vi "save DB after move.vi"(7 "Position (units) in":dbl, 8 "error in (no error)":errorcluster, 9 "Axis":i32, 10 "VISA resource name out in":refnum<visa-resource-name>, 11 "ESP302 in":refnum<class "ESP302.lvclass">) -> (0 "error out":errorcluster, 1 "Axis Status":T1(ring), 2 "VISA resource name out out":refnum<visa-resource-name>, 3 "ESP302 out":refnum<class "ESP302.lvclass">, 4 "Position (units) out":dbl)   [LabVIEW 2020, in "ESP302.lvclass"]
uses:
  ESP302/ESP302.lvclass
  ESP302/ESP302.lvclass/ESP302.ctl
  activeflag.ctl
  shared/OnOffTypeDef.ctl
  shared/CompressAndUpdate(Poly)/CompressAndUpdate(Enum).vi
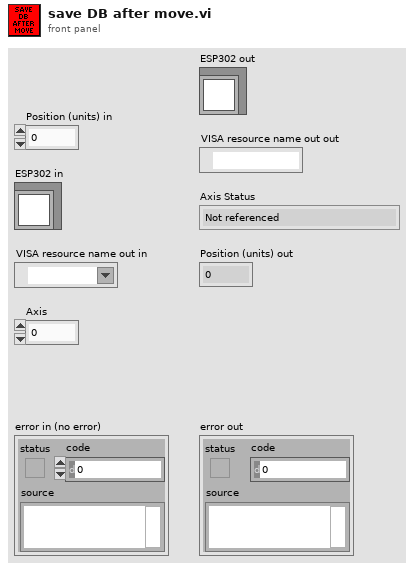
[diagram p1: front panel]
types:
  T1 = enum16{"Not referenced", "Homing", "Moving", "Ready"}
  T2 = typedef "activeflag.ctl" = enum16{"on", "off", "n/a"}
  T3 = typedef "OnOffTypeDef.ctl" = enum16{"off", "on"}
  T4 = typedef "ESP301.lvclass/SettingsTypdef.ctl" = cluster{"devport":string, "Position":cluster{"Axis 1":cluster{"Value":dbl, "Min":dbl, "Max":dbl, "StepSize":dbl, "Tolerance":dbl, "ValueActual":dbl}, "Axis 2":cluster{"Value":dbl, "Min":dbl, "Max":dbl, "StepSize":dbl, "Tolerance":dbl, "ValueActual":dbl}, "Axis 3":cluster{"Value":dbl, "Min":dbl, "Max":dbl, "StepSize":dbl, "Tolerance":dbl, "ValueActual":dbl}}, "Power":cluster{"Axis 1":T3, "Axis 2":T3, "Axis 3":T3}, "Status":cluster{"Axis 1":T5, "Axis 2":T5, "Axis 3":T5}, "Backlash":cluster{"Axis 1":cluster{"Value":dbl, "Min":dbl, "Max":dbl, "StepSize":dbl, "Tolerance":dbl, "ValueActual":dbl}, "Axis 2":cluster{"Value":dbl, "Min":dbl, "Max":dbl, "StepSize":dbl, "Tolerance":dbl, "ValueActual":dbl}, "Axis 3":cluster{"Value":dbl, "Min":dbl, "Max":dbl, "StepSize":dbl, "Tolerance":dbl, "ValueActual":dbl}}, "Home":cluster{"Axis 1":cluster{"Value":dbl, "Min":dbl, "Max":dbl, "StepSize":dbl, "Tolerance":dbl, "ValueActual":dbl}, "Axis 2":cluster{"Value":dbl, "Min":dbl, "Max":dbl, "StepSize":dbl, "Tolerance":dbl, "ValueActual":dbl}, "Axis 3":cluster{"Value":dbl, "Min":dbl, "Max":dbl, "StepSize":dbl, "Tolerance":dbl, "ValueActual":dbl}}, "MoveToHardLimit":cluster{"Axis 1":T6, "Axis 2":T6, "Axis 3":T6}, "relativeMove":cluster{"Axis 1neg":T3, "Axis 2neg":T3, "Axis 3neg":T3, "Axis 1pos":T3, "Axis 2pos":T3, "Axis 3pos":T3}, "stepsize":cluster{"Value":dbl, "Min":dbl, "Max":dbl, "StepSize":dbl, "Tolerance":dbl, "ValueActual":dbl}, "automotoroff":T3, "ResetBeforeMove":T3, "Enable":cluster{"Axis 1":T3, "Axis 2":T3, "Axis 3":T3}, "InitWithDBValues":T3}
  T5 = typedef "status_TypDef.ctl" = enum16{"Not referenced", "Homing", "Moving", "Ready"}
  T6 = typedef "Hardware limit.ctl" = enum16{"pos", "neg"}
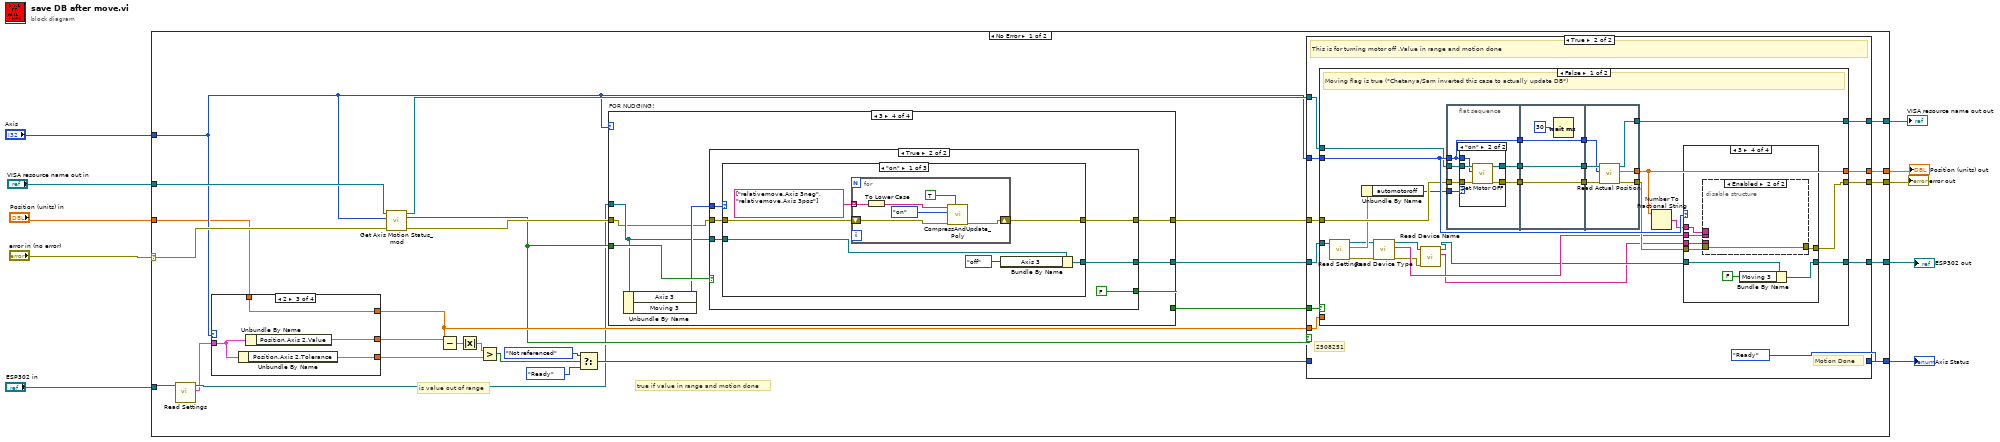
[diagram p0: block diagram]
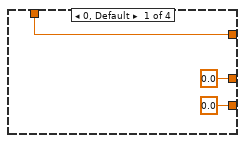
[diagram p2: hidden frame]
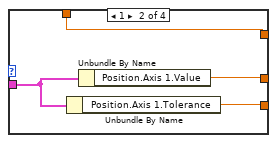
[diagram p3: hidden frame]
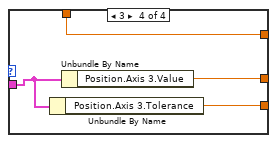
[diagram p4: hidden frame]
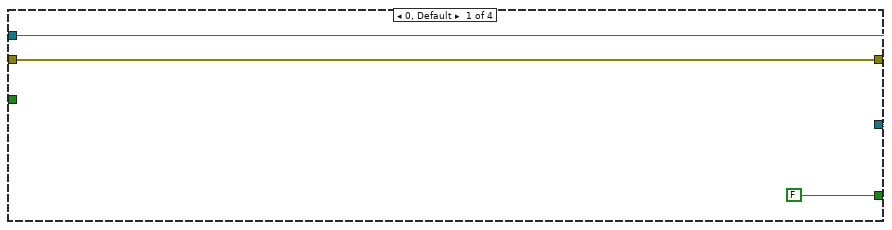
[diagram p5: hidden frame]
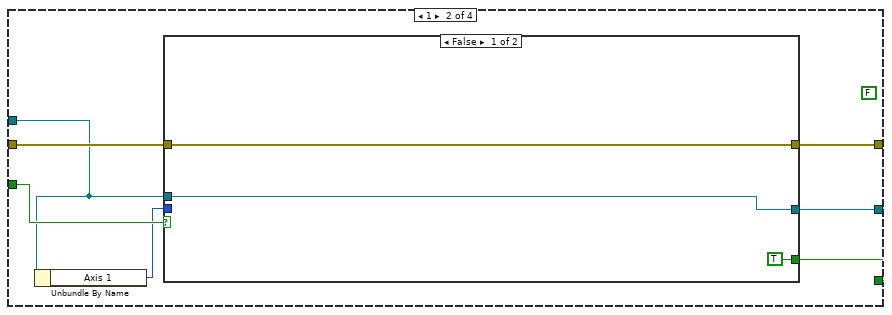
[diagram p6: hidden frame]
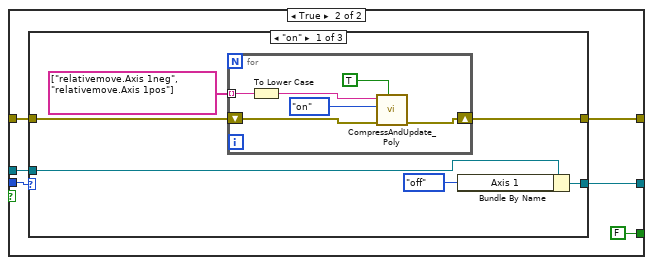
[diagram p7: hidden frame]
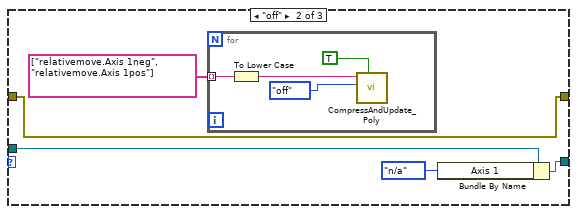
[diagram p8: hidden frame]
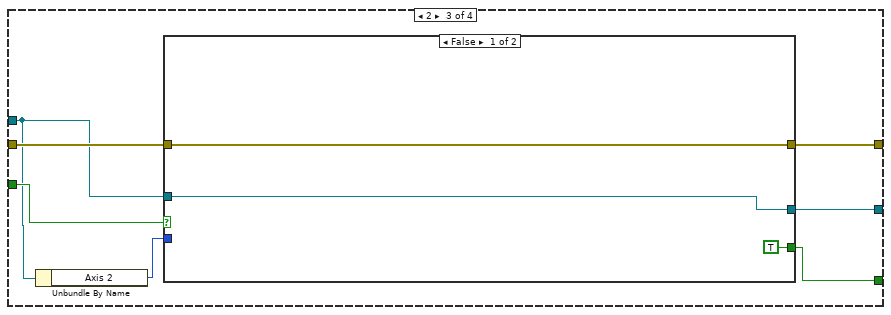
[diagram p10: hidden frame]
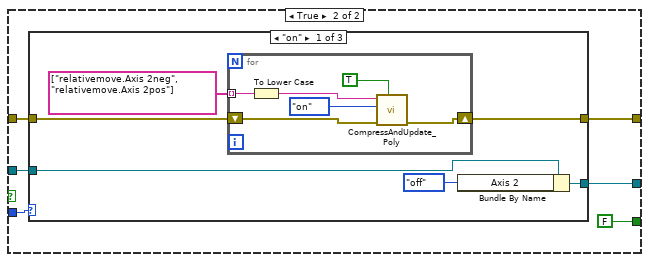
[diagram p11: hidden frame]
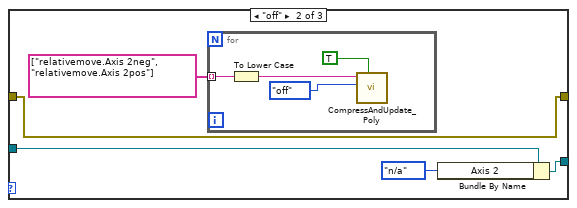
[diagram p12: hidden frame]
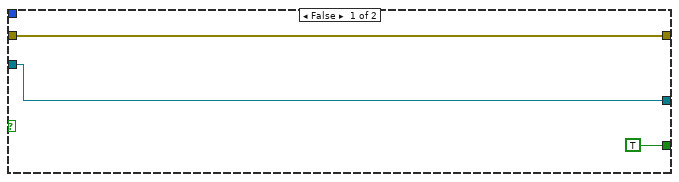
[diagram p14: hidden frame]
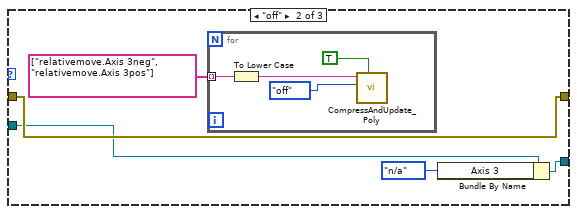
[diagram p15: hidden frame]
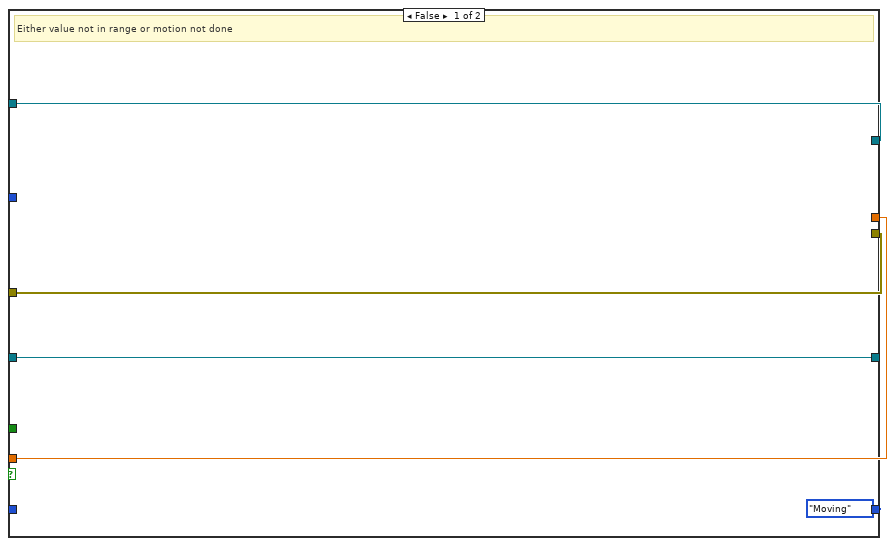
[diagram p17: hidden frame]
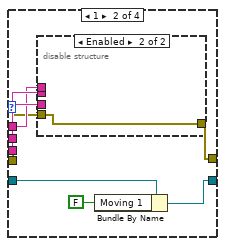
[diagram p20: hidden frame]
diagram:
  n1 = case shown="No Error" "error in (no error)" {
    selector: "error in (no error)" -> [w17 w288]
    tunnel: [w37 _] -> w4
    tunnel: [w36 w290] -> w3
    tunnel: [w35 _] -> w1
    tunnel: [w32 w289] -> w2
    tunnel: [w31 w288] -> w5
    tunnel: "ESP302 in" -> [w13 w289]
    tunnel: "VISA resource name out in" -> [w18 w290]
    tunnel: "Axis" -> [w16 _]
    tunnel: "Position (units) in" -> [w15 _]
    frame No Error {
      # "true if value in range and motion done"
      # "is value out of range"
      # "2508251"
      n2 = call-dynamic "Read Settings.vi"("ESP301 in"=w13) -> ("Settings"=w11:T4, "ESP301 out"=w14:refnum<class "ESP302.lvclass">)  [unwired: 8 in, 1 out]
      n3 = case shown="2" w16 {
        tunnel: [0.0 ("Tolerance") w44 w47 w51] -> w24
        tunnel: [0.0 ("Value") w43 w48 w52] -> w25
        tunnel: [w38 w42 w46 w50] -> w20
        tunnel: w15 -> [w38 w42 w46 w50]
        tunnel: w11 -> [_ w41 w45 w49]
        frame 0, Default {
        }
        frame 1 {
          n4 = Unbundle By Name(w41) -> ("Position.Axis 1.Tolerance"=w44:dbl)
          n5 = Unbundle By Name(w41) -> ("Position.Axis 1.Value"=w43:dbl)
        }
        frame 2 {
          n6 = Unbundle By Name(w45) -> ("Position.Axis 2.Tolerance"=w47:dbl)
          n7 = Unbundle By Name(w45) -> ("Position.Axis 2.Value"=w48:dbl)
        }
        frame 3 {
          n8 = Unbundle By Name(w49) -> ("Position.Axis 3.Tolerance"=w51:dbl)
          n9 = Unbundle By Name(w49) -> ("Position.Axis 3.Value"=w52:dbl)
        }
      }
      n10 = call "Get Axis Motion Status_mod.vi"("error in (no error)"=w17, "Axis (1)"=w16, "VISA resource name"=w18) -> ("error out"=w21:errorcluster, "Motion Done"=w19:bool, "VISA resource name out"=w23:refnum<visa-resource-name>)  [unwired: 2 in]
      n11 = Subtract(x=w25, y=w20) -> (x-y=w28:dbl)
      n12 = Absolute Value(x=w28) -> (abs(x)=w30:dbl)
      n13 = Greater?(x=w30, y=w24) -> (0:w26:bool)
      n14 = Select(t=T1."Not referenced" ("Axis 3"), s=w26, f=T1."Ready" ("Axis 3")) -> (s? t:f=w27:T1)
      n15 = case "FOR NUDGING!" shown="3" w16 {
        tunnel: w14 -> [w53 w58 w97 w136]
        tunnel: [FALSE ("Moving 3") w56 w95 w134] -> w34
        tunnel: w19 -> [_ w62 w101 w140]
        tunnel: [w53 w57 w96 w138] -> w33
        tunnel: w21 -> [w54 w60 w100 w135]
        tunnel: [w54 w59 w99 w139] -> w22
        frame 0, Default {
        }
        frame 1 {
          (unwired) FALSE ("Moving 2")
          n16 = Unbundle By Name(w58) -> ("Axis 1"=w61:T2)
          n17 = case shown="False" w62 {
            tunnel: [w65 w71] -> w57
            tunnel: [w64 w70] -> w59
            tunnel: w60 -> [w64 w69]
            tunnel: w58 -> [w65 w68]
            tunnel: w61 -> [_ w67]
            tunnel: [TRUE ("Moving 2") FALSE ("Moving 2")] -> w56
            frame False {
            }
            frame True {
              n18 = case shown="\"on\"" w67 {
                tunnel: [w76 w87 w93] -> w71
                tunnel: [w72 w84 w94] -> w70
                tunnel: w69 -> [w73 w84 w94]
                tunnel: w68 -> [w74 w85 w93]
                frame "on" {
                  n19 = for {
                    tunnel: string[] ["relativemove.Axis 1neg", "relativemove.Axis 1pos"] -> [w80] mode=indexing
                    shift-right: [w78] -> w72
                    shift-left: w73 -> [w79]
                    n20 = To Lower Case(string=w80) -> (all lower case string=w82:string)
                    n21 = call-poly "CompressAndUpdate_Poly.vi"("force CVT update (false)"=TRUE, "error in"=w79, "enum variant"=OnOffTypeDef."on" ("Axis 1neg"), "command or variable name"=w82) -> ("error out"=w78:errorcluster)  [unwired: 7 in]
                  }
                  n22 = Bundle By Name(cluster=w74, "Axis 1"=activeflag."off" ("ActiveFlag")) -> (w76:refnum<class "ESP302.lvclass">)
                }
                frame "off" {
                  n23 = for {
                    tunnel: string[] ["relativemove.Axis 1neg", "relativemove.Axis 1pos"] -> [w89] mode=indexing
                    n24 = To Lower Case(string=w89) -> (all lower case string=w91:string)
                    n25 = call-poly "CompressAndUpdate_Poly.vi"("force CVT update (false)"=TRUE, "enum variant"=OnOffTypeDef."off" ("Axis 1neg"), "command or variable name"=w91) -> ()  [unwired: 8 in, 1 out]
                  }
                  n26 = Bundle By Name(cluster=w85, "Axis 1"=activeflag."n/a" ("ActiveFlag")) -> (w87:refnum<class "ESP302.lvclass">)
                }
                frame "n/a", Default {
                }
              }
            }
          }
        }
        frame 2 {
          n27 = Unbundle By Name(w97) -> ("Axis 2"=w98:T2)
          n28 = case shown="False" w101 {
            tunnel: [w104 w110] -> w96
            tunnel: [w103 w109] -> w99
            tunnel: w100 -> [w103 w108]
            tunnel: w97 -> [w104 w107]
            tunnel: w98 -> [_ w106]
            tunnel: [TRUE ("Moving 2") FALSE ("Moving 2")] -> w95
            frame False {
            }
            frame True {
              n29 = case shown="\"on\"" w106 {
                tunnel: [w115 w126 w132] -> w110
                tunnel: [w111 w123 w133] -> w109
                tunnel: w108 -> [w112 w123 w133]
                tunnel: w107 -> [w113 w124 w132]
                frame "on" {
                  n30 = for {
                    tunnel: string[] ["relativemove.Axis 2neg", "relativemove.Axis 2pos"] -> [w119] mode=indexing
                    shift-right: [w117] -> w111
                    shift-left: w112 -> [w118]
                    n31 = To Lower Case(string=w119) -> (all lower case string=w121:string)
                    n32 = call-poly "CompressAndUpdate_Poly.vi"("force CVT update (false)"=TRUE, "error in"=w118, "enum variant"=OnOffTypeDef."on" ("Axis 1neg"), "command or variable name"=w121) -> ("error out"=w117:errorcluster)  [unwired: 7 in]
                  }
                  n33 = Bundle By Name(cluster=w113, "Axis 2"=activeflag."off" ("ActiveFlag")) -> (w115:refnum<class "ESP302.lvclass">)
                }
                frame "off" {
                  n34 = for {
                    tunnel: string[] ["relativemove.Axis 2neg", "relativemove.Axis 2pos"] -> [w128] mode=indexing
                    n35 = To Lower Case(string=w128) -> (all lower case string=w130:string)
                    n36 = call-poly "CompressAndUpdate_Poly.vi"("force CVT update (false)"=TRUE, "enum variant"=OnOffTypeDef."off" ("Axis 1neg"), "command or variable name"=w130) -> ()  [unwired: 8 in, 1 out]
                  }
                  n37 = Bundle By Name(cluster=w124, "Axis 2"=activeflag."n/a" ("ActiveFlag")) -> (w126:refnum<class "ESP302.lvclass">)
                }
                frame "n/a", Default {
                }
              }
            }
          }
        }
        frame 3 {
          n38 = Unbundle By Name(w136) -> ("Axis 3"=w137:T2)  [unwired: 1 out]
          n39 = case shown="True" w140 {
            tunnel: [w142 w145] -> w138
            tunnel: [w143 w149] -> w139
            tunnel: w135 -> [w143 w148]
            tunnel: w137 -> [_ w147]
            tunnel: w136 -> [w142 w146]
            tunnel: [TRUE ("Moving 2") FALSE ("Moving 2")] -> w134
            frame False {
            }
            frame True {
              n40 = case shown="\"on\"" w147 {
                tunnel: [w154 w165 w171] -> w145
                tunnel: [w151 w163 w172] -> w149
                tunnel: w148 -> [w152 w163 w172]
                tunnel: w146 -> [w150 w162 w171]
                frame "on" {
                  n41 = for {
                    tunnel: string[] ["relativemove.Axis 3neg", "relativemove.Axis 3pos"] -> [w158] mode=indexing
                    shift-right: [w156] -> w151
                    shift-left: w152 -> [w157]
                    n42 = To Lower Case(string=w158) -> (all lower case string=w160:string)
                    n43 = call-poly "CompressAndUpdate_Poly.vi"("force CVT update (false)"=TRUE, "error in"=w157, "enum variant"=OnOffTypeDef."on" ("Axis 1neg"), "command or variable name"=w160) -> ("error out"=w156:errorcluster)  [unwired: 7 in]
                  }
                  n44 = Bundle By Name(cluster=w150, "Axis 3"=activeflag."off" ("ActiveFlag")) -> (w154:refnum<class "ESP302.lvclass">)
                }
                frame "off" {
                  n45 = for {
                    tunnel: string[] ["relativemove.Axis 3neg", "relativemove.Axis 3pos"] -> [w167] mode=indexing
                    n46 = To Lower Case(string=w167) -> (all lower case string=w169:string)
                    n47 = call-poly "CompressAndUpdate_Poly.vi"("force CVT update (false)"=TRUE, "enum variant"=OnOffTypeDef."off" ("Axis 1neg"), "command or variable name"=w169) -> ()  [unwired: 8 in, 1 out]
                  }
                  n48 = Bundle By Name(cluster=w162, "Axis 3"=activeflag."n/a" ("ActiveFlag")) -> (w165:refnum<class "ESP302.lvclass">)
                }
                frame "n/a", Default {
                }
              }
            }
          }
        }
      }
      n49 = case shown="True" w19 {
        tunnel: [T1."Moving" ("Axis 3") T1."Ready" ("Axis 3")] -> w35
        tunnel: w20 -> [w173 w183]
        tunnel: w33 -> [w176 w181]
        tunnel: w16 -> [_ w180]
        tunnel: [w176 w188] -> w32
        tunnel: w23 -> [w175 w187]
        tunnel: w22 -> [w174 w186]
        tunnel: [w175 w185] -> w36
        tunnel: [w174 w184] -> w31
        tunnel: [w173 w182] -> w37
        tunnel: w34 -> [_ w179]
        tunnel: w27 -> [_ _]
        frame False {
          # "Either value not in range or motion not done"
        }
        frame True {
          # "Motion Done"
          # "This is for turning motor off .Value in range and motion done"
          n50 = case shown="False" w179 {
            tunnel: w180 -> [w212 _]
            tunnel: w181 -> [w196 w287]
            tunnel: [w213 w287] -> w188
            tunnel: w187 -> [w211 w286]
            tunnel: w186 -> [w210 w285]
            tunnel: [w209 w286] -> w185
            tunnel: [w199 w285] -> w184
            tunnel: w183 -> [_ w284]
            tunnel: [w201 w284] -> w182
            frame False {
              # "Moving flag is true (*Chetanya/Sam inverted this case to actually update DB*)"
              n51 = call-dynamic "Read Settings.vi"("ESP301 in"=w196) -> ("error out"=w189:errorcluster, "Settings"=w198:T4, "ESP301 out"=w195:refnum<class "ESP302.lvclass">)  [unwired: 8 in]
              n52 = Unbundle By Name(w198) -> ("automotoroff"=w197:T3)
              n53 = call-dynamic "Read Device Type.vi"("error in (no error)"=w189, "ESP301 in"=w195) -> ("error out"=w191:errorcluster, "Device Type"=w194:string, "ESP301 out"=w193:refnum<class "ESP302.lvclass">)  [unwired: 7 in]
              n54 = call-dynamic "Read Device Name.vi"("error in (no error)"=w191, "ESP301 in"=w193) -> ("Device Name"=w190:string, "ESP301 out"=w192:refnum<class "ESP302.lvclass">)  [unwired: 7 in, 1 out]
              n55 = flat-sequence {
                tunnel: w212 -> [w215]
                tunnel: w211 -> [w219]
                tunnel: w210 -> [w218]
                tunnel: [w217] -> w208
                tunnel: [w216] -> w206
                tunnel: [w215] -> w204
                tunnel: w197 -> [w214]
                tunnel: w208 -> [w230]
                tunnel: [w230] -> w207
                tunnel: w206 -> [w229]
                tunnel: [w229] -> w205
                tunnel: w204 -> [w227]
                tunnel: [w227] -> w203
                tunnel: [w231] -> w200
                tunnel: [w232] -> w209
                tunnel: w207 -> [w235]
                tunnel: w205 -> [w236]
                tunnel: w203 -> [w234]
                tunnel: [w233] -> w201
                frame #0 {
                  n56 = case shown="\"on\"" w214 {
                    tunnel: w219 -> [w221 w226]
                    tunnel: w218 -> [w220 w225]
                    tunnel: [w221 w224] -> w217
                    tunnel: [w220 w223] -> w216
                    tunnel: w215 -> [_ w222]
                    frame "off", Default {
                    }
                    frame "on" {
                      n57 = call "Set Motor OFF.vi"("error in (no error)"=w225, "Axis (1)"=w222, "VISA resource name"=w226) -> ("error out"=w223:errorcluster, "VISA resource name out"=w224:refnum<visa-resource-name>)  [unwired: 3 in]
                    }
                  }
                }
                frame #1 {
                  n58 = Wait (ms)(milliseconds to wait=u32 30) -> ()  [unwired: 1 out]
                }
                frame #2 {
                  n59 = call "Read Actual Position.vi"("error in (no error)"=w236, "Axis (1)"=w234, "VISA resource name"=w235) -> ("error out"=w231:errorcluster, "Position (units)"=w233:dbl, "VISA resource name out"=w232:refnum<visa-resource-name>)  [unwired: 2 in]
                }
              }
              n60 = Number To Fractional String(number=w201) -> (F-format string=w202:string)  [unwired: 3 in]
              n61 = case shown="3" w212 {
                tunnel: w192 -> [w238 w245 w260 w275]
                tunnel: [w238 w246 w261 w276] -> w213
                tunnel: w194 -> [_ w243 w257 w272]
                tunnel: w190 -> [_ w242 w258 w273]
                tunnel: w202 -> [_ w241 w256 w271]
                tunnel: w200 -> [w237 w240 w255 w270]
                tunnel: [w237 w239 w254 w269] -> w199
                frame 0, Default {
                }
                frame 1 {
                  n62 = disable-structure shown="Enabled" {
                    disable-tunnel: w243 -> [w252 _]
                    disable-tunnel: w242 -> [w251 _]
                    disable-tunnel: w241 -> [w250 _]
                    disable-tunnel: w240 -> [w248 w253]
                    disable-tunnel: [w247 w253] -> w239
                    frame Disabled {
                      n63 = call "Update Variable.vi"("Device Type"=w252, "error in (no error)"=w248, "device name"=w251, "Variable Value"=w250, "Variable Name"="Position.Axis 1" ("Variable Value")) -> ("error out"=w247:errorcluster)  [unwired: 6 in]
                    }
                    frame Enabled {
                    }
                  }
                  n64 = Bundle By Name(cluster=w245, "Moving 1"=FALSE) -> (w246:refnum<class "ESP302.lvclass">)
                }
                frame 2 {
                  n65 = disable-structure shown="Enabled" {
                    disable-tunnel: w258 -> [w267 _]
                    disable-tunnel: w257 -> [w266 _]
                    disable-tunnel: w256 -> [w264 _]
                    disable-tunnel: w255 -> [w263 w268]
                    disable-tunnel: [w262 w268] -> w254
                    frame Disabled {
                      n66 = call "Update Variable.vi"("Device Type"=w266, "error in (no error)"=w263, "device name"=w267, "Variable Value"=w264, "Variable Name"="Position.Axis 2" ("Variable Value")) -> ("error out"=w262:errorcluster)  [unwired: 6 in]
                    }
                    frame Enabled {
                    }
                  }
                  n67 = Bundle By Name(cluster=w260, "Moving 2"=FALSE ("Moving 1")) -> (w261:refnum<class "ESP302.lvclass">)
                }
                frame 3 {
                  n68 = disable-structure shown="Enabled" {
                    disable-tunnel: w273 -> [w282 _]
                    disable-tunnel: w272 -> [w281 _]
                    disable-tunnel: w271 -> [w279 _]
                    disable-tunnel: w270 -> [w278 w283]
                    disable-tunnel: [w277 w283] -> w269
                    frame Disabled {
                      n69 = call "Update Variable.vi"("Device Type"=w281, "error in (no error)"=w278, "device name"=w282, "Variable Value"=w279, "Variable Name"="Position.Axis 3" ("Variable Value")) -> ("error out"=w277:errorcluster)  [unwired: 6 in]
                    }
                    frame Enabled {
                    }
                  }
                  n70 = Bundle By Name(cluster=w275, "Moving 3"=FALSE ("Moving 1")) -> (w276:refnum<class "ESP302.lvclass">)
                }
              }
            }
            frame True {
              # "Moving flag is false, no need to turn off motor since should already be false."
            }
          }
        }
      }
    }
    frame Error {
    }
  }
  "Position (units) out" <- w4
  "error out" <- w5
  "VISA resource name out out" <- w3
  "ESP302 out" <- w2
  "Axis Status" <- w1
